vi "SVT Build Result Table (1 Ch).vi"(0 "octave spectrum":T5 {"band power" format="%.2f"; "nominal frequencies [Hz]" format="%.2f"}, 5 "precision (1)":i16=1 min=0, 9 "octave info":T1={"standard"=enum."ANSI S1.11", "bandwidth"=enum."1 octave", "low band"=0, "high band"=0, "weighting filter"=0, "dB reference"=0.0, "dB On"=FALSE, "unit label"="", "channel name"="", "description"="", "engineering units"=1, "custom label"="", "spectrum type"=enum."magnitude", "spectral density"=FALSE, "filters settled"=FALSE} {"engineering units" items=["custom..."=0, "V"=1, "A"=21, "C"=30, "pC"=31, "s"=32, "-"=29, "Pa"=2, "N"=20, "g"=3, "m/s^2"=4, "m/s"=5, "m"=6, "mm/s"=12, "mm"=13, "micron/s"=14, "micron"=15, "in/s^2"=7, "in/s"=8, "in"=9, "mil/s"=10, "mil"=11, "rad/s^2"=16, "rad/s"=17, "rad"=18, "deg/s^2"=26, "deg/s"=27, "deg"=28, "RPM"=22, "cycle/s^2"=23, "Hz"=24, "cycle"=25, "strain"=19]; "dB reference" format="%.2e"; "weighting filter" items=["Linear", "A-weighting", "B-weighting", "C-weighting", "ITU-R 468-4", "Dolby", "CCITT", "C-message", "Wb", "Wc", "Wd", "We", "Wf", "Wh", "Wj", "Wk", "Wm", "AES17 20 kHz lowpass", "AES17 40 kHz lowpass", "AES17 20 kHz highpass", "AES17 40 kHz highpass"]}, 11 "error in (no error)":errorcluster, 12 "include units with values (T)":bool=TRUE) -> (4 "result table":string[][](table), 6 "column headers":string[](array[string]), 15 "error out":errorcluster)   [LabVIEW 2017, in "SoundVib_Octave.lvlib"]
doc: "Generates a table of the results of a fractional-octave analysis. The first column of the table contains the nominal frequencies in Hz. The second and subsequent columns contain the 1/n band power with the appropriate unit label. Wire data to the <B>octave spectrum</B> input to determine the polymorphic instance to use or manually select the instance."
uses:
  <vilib>/addons/Sound and Vibration/svt_Octave/SoundVib_Octave.lvlib
  <vilib>/addons/_NISVFA/_Shared subVIs/Controls/svc_Octave Info.ctl
  <vilib>/addons/_NISVFA/_Shared subVIs/Controls/svc_Octave Standard.ctl
  <vilib>/addons/_NISVFA/_Shared subVIs/Controls/svc_Weighting Filter Text Ring.ctl
  <vilib>/addons/_NISVFA/_Shared subVIs/Controls/svc_Engineering Units Text Ring.ctl
  <vilib>/addons/_NISVFA/_Shared subVIs/Common/svc_Sort XY Results.vi
  <vilib>/addons/Sound and Vibration/svt_Octave_2014 standard/SoundVib_Octave_2014 standard.lvlib
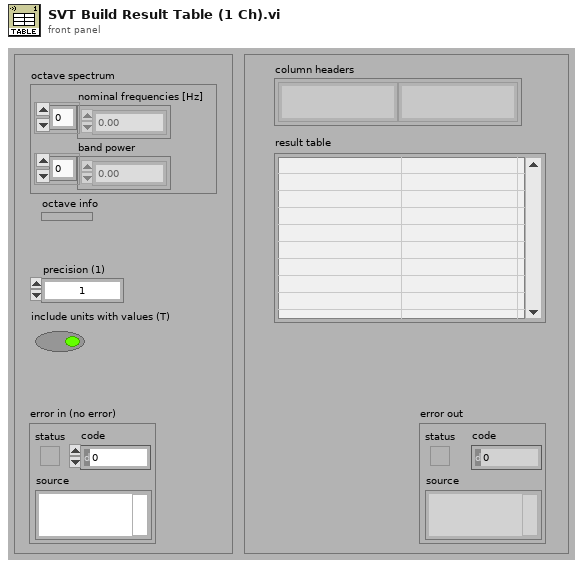
[diagram p1: front panel]
types:
  T1 = typedef "svc_Octave Info.ctl" = cluster{"standard":T2, "bandwidth":enum16{"1 octave", "1/3 octave", "1/6 octave", "1/12 octave", "1/24 octave"}, "low band":i32, "high band":i32, "weighting filter":T3, "dB reference":dbl, "dB On":bool, "unit label":string, "channel name":string, "description":string, "engineering units":T4, "custom label":string, "spectrum type":enum16{"power", "magnitude"}, "spectral density":bool, "filters settled":bool}
  T2 = typedef "svc_Octave Standard.ctl" = enum16{"ANSI S1.11", "IEC 61260"}
  T3 = typedef "svc_Weighting Filter Text Ring.ctl" = u16
  T4 = typedef "svc_Engineering Units Text Ring.ctl" = u16
  T5 = cluster{"nominal frequencies [Hz]":dbl[], "band power":dbl[]}
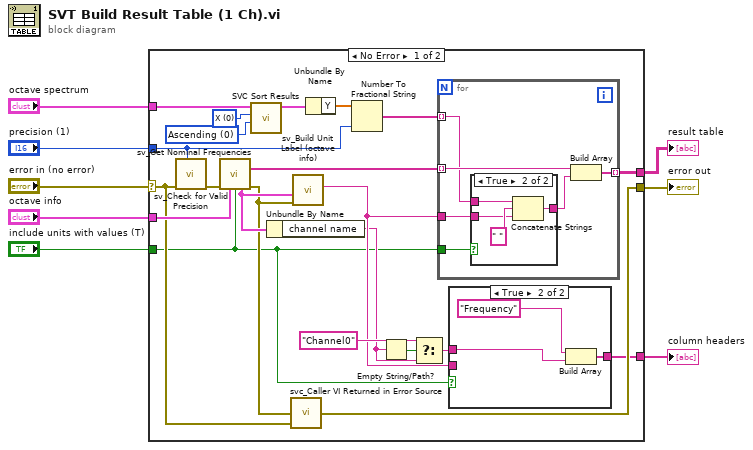
[diagram p0: block diagram]
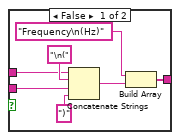
[diagram p2: hidden frame]
diagram:
  n1 = case shown="No Error" "error in (no error)" {
    selector: "error in (no error)" -> [w25 w52]
    tunnel: [w28 w52] -> w8
    tunnel: "precision (1)" -> [w10 _]
    tunnel: [w30 _] -> w6
    tunnel: "octave spectrum" -> [w15 _]
    tunnel: "octave info" -> [w26 _]
    tunnel: "include units with values (T)" -> [w16 _]
    tunnel: [w21 _] -> w1
    frame No Error {
      w12 = u16 0 items=["Ascending", "Descending"] ("sort order")
      w13 = u16 0 items=["X", "Y"] ("sort by")
      n2 = call <vilib>:"sv_Check for Valid Precision.vi"("precision (1)"=w10, "error in (no error)"=w25) -> ("error out"=w27:errorcluster)  [unwired: 9 in]
      n3 = call <vilib>:"sv_Get Nominal Frequencies.vi"("error in (no error)"=w27, "octave info"=w26, "include units (T)"=w16) -> ("nominal frequencies (string)"=w29:string[], "dup octave info"=w20:T1, "error out"=w17:errorcluster)  [unwired: 10 in]
      n4 = call-poly <vilib>:"SVC Sort Results.vi"("sort order"=w12, "sort by"=w13, "XY in"=w15) -> ("sorted XY"=w14:cluster{"X":dbl[], "Y":dbl[]})  [unwired: 7 in, 1 out]
      n5 = Unbundle By Name(w20) -> ("channel name"=w18:string)
      n6 = call <vilib>:"svc_Caller VI Returned in Error Source.vi"("warning input to caller"=w25, "error in (no error)"=w17) -> ("error out"=w28:errorcluster)  [unwired: 3 in]
      n7 = call <vilib>:"sv_Build Unit Label (octave info).vi"("error in (no error)"=w17, "octave info"=w20) -> ("unit label"=w19:string)  [unwired: 7 in, 2 out]
      n8 = Unbundle By Name(w14) -> ("Y"=w11:dbl[])
      n9 = Number To Fractional String(number=w11, precision (6)=w10) -> (F-format string=w9:string[])  [unwired: 2 in]
      n10 = Empty String/Path?(string/path=w18) -> (empty?=w22:bool)
      n11 = Select(t="Channel0", s=w22, f=w18) -> (s? t:f=w23:string)
      n12 = for {
        tunnel: w29 -> [w46] mode=indexing
        tunnel: [w45] -> w30 mode=indexing
        tunnel: w16 -> [w43]
        tunnel: w19 -> [w42]
        tunnel: w9 -> [w41] mode=indexing
        n13 = case shown="True" w43 {
          tunnel: [w47 w51] -> w44
          tunnel: w41 -> [w47 w49]
          tunnel: w42 -> [_ w48]
          frame False {
          }
          frame True {
            n14 = Concatenate Strings(w49, " ", w48) -> (w51:string)
          }
        }
        n15 = Build Array(w46, w44) -> (w45:string[])
      }
      n16 = case shown="True" w16 {
        tunnel: w23 -> [w35 w38]
        tunnel: [w32 w39] -> w21
        tunnel: w19 -> [w31 _]
        frame False {
          n17 = Concatenate Strings(w35, "\n(" ("string"), w31, ")" ("string")) -> (w34:string)
          n18 = Build Array("Frequency\n(Hz)", w34) -> (w32:string[])
        }
        frame True {
          n19 = Build Array("Frequency", w38) -> (w39:string[])
        }
      }
    }
    frame Error {
    }
  }
  "error out" <- w8
  "result table" <- w6
  "column headers" <- w1
